vi "Create Output Folder (SubVI).vi"(8 "Settings File Name":path=path "C:/MWT/Config.ini", 11 "DLL Input Param":T1={"DateTimeStamp"="DateTimeStamp", "Genotype 1"="genotype1", "Genotype 2"="genotype2", "Rig Name"="stimulationMode", "STIM Mode"="t21", "Light Intensity (%)"=100, "Pixel Resolution (um/pixel)"=100.0, "Gamma"=0.2, "Yoked File Name"="none", "Yoked File Enable"=FALSE, "Output Folder Name"=path "", "Frame Number"=0, "Time Stamp (us)"=0, "Exp STOP"=0, "Contour"=[], "SPINE"=[], "Larvae ID"=[], "Larvae Valid?"=[], "Image Height"=0, "Image Width"=0, "Pixel Intensity Low"=0, "Pixel Intensity High"=0, "Box Side Low"=0, "Box Side High"=0, "Box W+L Low"=0, "Box W+L High"=0, "Area Low"=0, "Area High"=0, "N SPINE"=0, "BG SUB TH"=0, "Min Contour Points"=0, "STIM Array"=[], "Stimulus Label Array"=[], "Flip Laravae ID"=[], "IR Intensity"=0}) -> (3 "Folder Name":path)   [LabVIEW 2020]
uses:
  Controls (HOST)/File Name Prefix.ctl
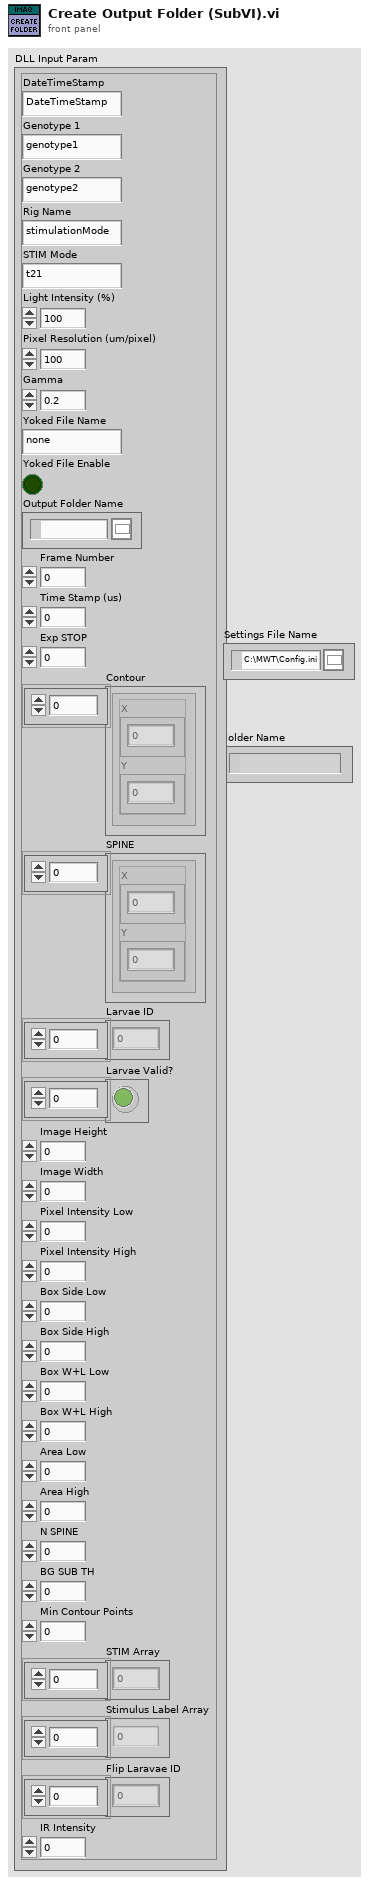
[diagram p1: front panel]
types:
  T1 = typedef "File Name Prefix.ctl" = cluster{"DateTimeStamp":string, "Genotype 1":string, "Genotype 2":string, "Rig Name":string, "STIM Mode":string, "Light Intensity (%)":i32, "Pixel Resolution (um/pixel)":dbl, "Gamma":dbl, "Yoked File Name":string, "Yoked File Enable":bool, "Output Folder Name":path, "Frame Number":u64, "Time Stamp (us)":u64, "Exp STOP":i32, "Contour":cluster{"X":i32[], "Y":i32[]}[], "SPINE":cluster{"X":dbl[], "Y":dbl[]}[], "Larvae ID":u32[], "Larvae Valid?":bool[], "Image Height":i32, "Image Width":i32, "Pixel Intensity Low":i32, "Pixel Intensity High":i32, "Box Side Low":i32, "Box Side High":i32, "Box W+L Low":i32, "Box W+L High":i32, "Area Low":i32, "Area High":i32, "N SPINE":i32, "BG SUB TH":i32, "Min Contour Points":i32, "STIM Array":dbl[], "Stimulus Label Array":u8[], "Flip Laravae ID":i32[], "IR Intensity":i32}
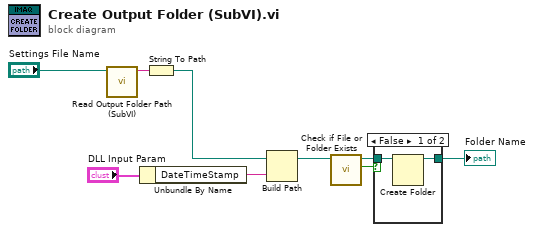
[diagram p0: block diagram]
diagram:
  n1 = call "Read Output Folder Path (SubVI).vi"("Settings File Name"="Settings File Name") -> ("Output Folder"=w3:string)  [unwired: 10 in]
  n2 = Unbundle By Name("DLL Input Param") -> ("DateTimeStamp"=w4:string)
  n3 = String To Path(string=w3) -> (path=w2:path)
  n4 = Build Path(base path=w2, name or relative path=w4) -> (appended path=w5:path)
  n5 = call <vilib>:"Check if File or Folder Exists.vi"("path"=w5) -> ("file or folder exists?"=w9:bool, "dup path"=w8:path)  [unwired: 8 in, 1 out]
  n6 = case shown="False" w9 {
    tunnel: w8 -> [w11 w12]
    tunnel: [w10 w12] -> w7
    frame False {
      n7 = Create Folder(path (use dialog)=w11) -> (created path=w10:path)  [unwired: 2 in, 2 out]
    }
    frame True {
    }
  }
  "Folder Name" <- w7
